vi "Wrapper.vi"(8 "error in (no error)":errorcluster, 10 "Actor in":refnum<class "Actor.lvclass">, 11 "Update gController Data MSG in":refnum<class "Update gController Data MSG.lvclass">) -> (0 "error out":errorcluster, 3 "gController out":refnum<class "gController.lvclass">)   [LabVIEW 2017, in "Controller.lvlib" / "Update gController Data MSG.lvclass"]
uses:
  Update gController Data MSG.lvclass
  C:/Program Files (x86)/National Instruments/LabVIEW 2017/vi.lib/MSR Consulting, LLC/General Reuse/Generic Update Data MSG/Generic Update Data MSG.lvclass
  gController.lvclass
  C:/Program Files (x86)/National Instruments/LabVIEW 2017/vi.lib/MSR Consulting, LLC/General Reuse/SuperActor/SuperActor.lvclass
  <vilib>/ActorFramework/Actor/Actor.lvclass
  gController.lvclass/gController.ctl
  <vilib>/MSR Consulting, LLC/General Reuse/SuperActor/SuperActor.lvclass/SuperActor.ctl
  <vilib>/MSR Consulting, LLC/General Reuse/Generic Update Data MSG/Generic Update Data MSG.lvclass/Generic Update Data MSG.ctl
  <vilib>/MSR Consulting, LLC/General Reuse/Generic Update Data MSG/Read Data.vi
  <vilib>/MSR Consulting, LLC/General Reuse/Generic Update Data MSG/Read ID.vi
  Read DataMap.vi
  <vilib>/MSR Consulting, LLC/General Reuse/SuperActor/Read Log Session.vi
  <vilib>/MSR Consulting, LLC/General Reuse/Data/Data.lvclass
  <vilib>/MSR Consulting, LLC/General Reuse/Session APIs/_Session Fwk/Session - Root.lvclass
  <vilib>/MSR Consulting, LLC/General Reuse/Session APIs/Session Log/System Log.lvclass
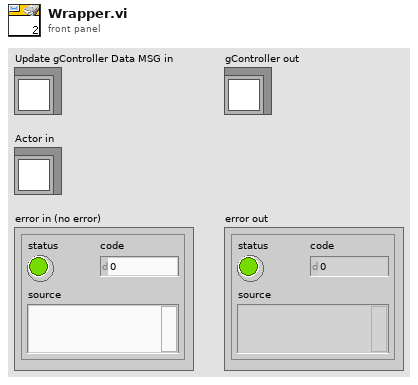
[diagram p1: front panel]
types:
  T1 = typedef "Session - Root.lvclass/Session Handle.ctl" = refnum<data-value>
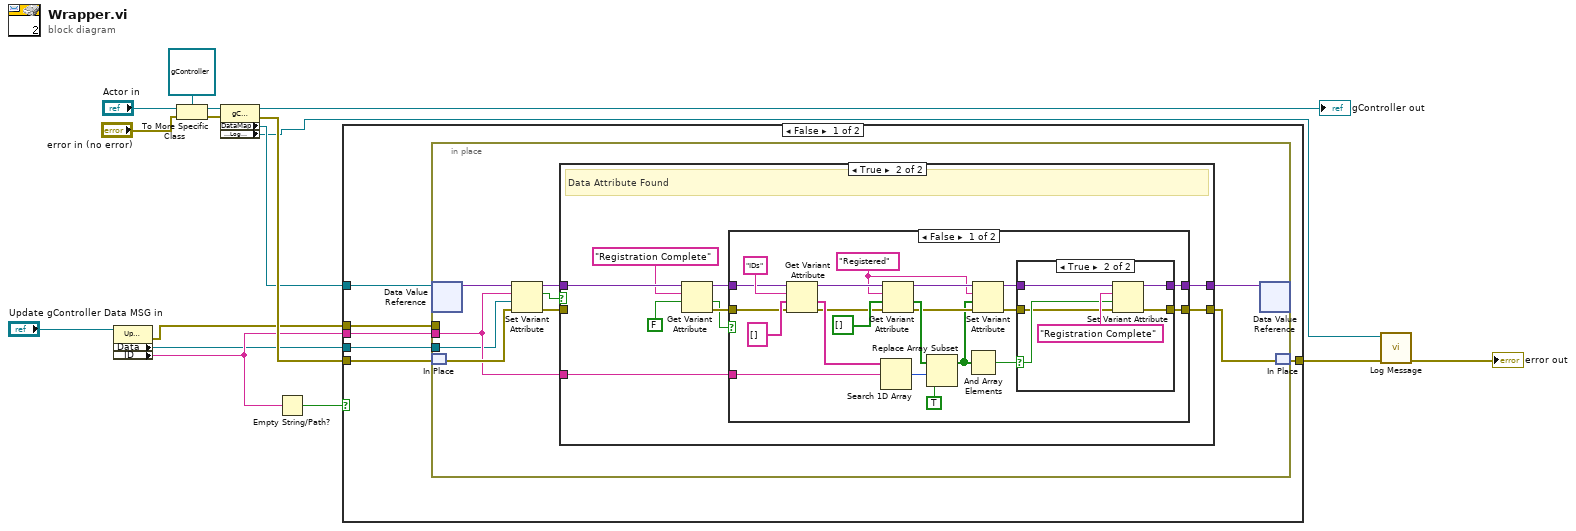
[diagram p0: block diagram]
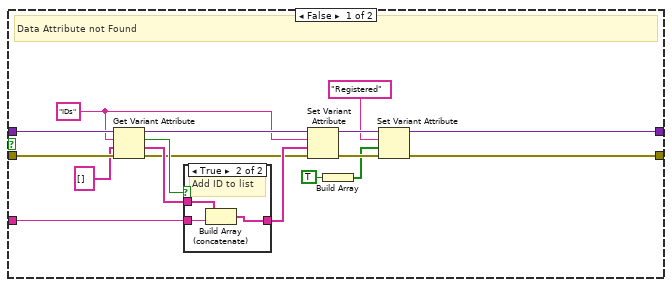
[diagram p2: hidden frame]
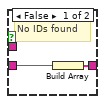
[diagram p3: hidden frame]
diagram:
  n1 = property class="Update gController Data MSG.lvc"(reference="Update gController Data MSG in") -> (error out=w5:errorcluster, "Data"=w4:refnum<class "Data.lvclass">, "ID"=w6:string)  [unwired: 1 in, 1 out]
  n2 = To More Specific Class(target class=refnum<class "gController.lvclass"> refnum ("Controller.lvlib:gController"), reference="Actor in", error in="error in (no error)") -> (specific class reference=w11:refnum<class "gController.lvclass">, error out=w15:errorcluster)
  n3 = property class="gController"(reference=w11, error in=w15) -> (reference out=→"gController out":refnum<class "gController.lvclass">, error out=w16:errorcluster, "DataMap"=w12:refnum<data-value>, "Accessors:Log Session"=w3:T1)
  n4 = Empty String/Path?(string/path=w6) -> (empty?=w8:bool)
  n5 = case shown="False" w8 {
    tunnel: [w22 w94] -> w2
    tunnel: w16 -> [w21 w94]
    tunnel: w6 -> [w20 _]
    tunnel: w5 -> [w19 _]
    tunnel: w12 -> [w18 _]
    tunnel: w4 -> [w17 _]
    frame False {
      n6 = in-place {
        in-place-border: w19 -> [_]
        in-place-border: w20 -> [w26]
        in-place-border: w17 -> [w23]
        n7 = in-place-dvr #1(w18) -> (w29:variant)  [unwired: 1 out]
        n8 = in-place-match #2(w21) -> (w27:errorcluster)
        n9 = Set Variant Attribute(Variant=w29, name=w26, value=w23, error in=w27) -> (Variant out=w31:variant, replaced=w30:bool, error out=w28:errorcluster)
        n10 = case shown="True" w30 {
          tunnel: w31 -> [w48 w60]
          tunnel: w26 -> [w47 w61]
          tunnel: [w45 w62] -> w24
          tunnel: w28 -> [w46 _]
          tunnel: [w44 w55] -> w25
          frame False {
            w41 = "IDs" ("name")
            # "Data Attribute not Found"
            n11 = Get Variant Attribute(Variant=w48, name=w41, default value (empty Variant)=string[] [], error in=w46) -> (duplicate Variant=w42:variant, found=w40:bool, value=w39:string[], error out=w37:errorcluster)
            n12 = case shown="True" w40 {
              tunnel: w39 -> [_ w53]
              tunnel: w47 -> [w50 w52]
              tunnel: [w49 w51] -> w38
              frame False {
                # "No IDs found"
                n13 = Build Array(w50) -> (w49:string[])
              }
              frame True {
                # "Add ID to list"
                n14 = Build Array (concatenate)(w53, w52) -> (w51:string[])
              }
            }
            n15 = Set Variant Attribute(Variant=w42, name=w41, value=w38, error in=w37) -> (Variant out=w36:variant, error out=w35:errorcluster)  [unwired: 1 out]
            n16 = Build Array(TRUE) -> (w32:bool[])
            n17 = Set Variant Attribute(Variant=w36, name="Registered", value=w32, error in=w35) -> (Variant out=w45:variant, error out=w44:errorcluster)  [unwired: 1 out]
          }
          frame True {
            # "Data Attribute Found"
            n18 = Get Variant Attribute(Variant=w60, name="Registration Complete", default value (empty Variant)=FALSE) -> (duplicate Variant=w57:variant, value=w54:bool, error out=w56:errorcluster)  [unwired: 1 in, 1 out]
            n19 = case shown="False" w54 {
              tunnel: [w66 w93] -> w62
              tunnel: w61 -> [w80 _]
              tunnel: w57 -> [w78 w93]
              tunnel: w56 -> [w77 w92]
              tunnel: [w64 w92] -> w55
              frame False {
                w69 = "Registered" ("name")
                n20 = Get Variant Attribute(Variant=w78, name="IDs", default value (empty Variant)=string[] [], error in=w77) -> (duplicate Variant=w79:variant, value=w81:string[], error out=w63:errorcluster)  [unwired: 1 out]
                n21 = Search 1D Array(1D array=w81, element=w80) -> (index of element=w74:i32)  [unwired: 1 in]
                n22 = Get Variant Attribute(Variant=w79, name=w69, default value (empty Variant)=bool[] [], error in=w63) -> (duplicate Variant=w72:variant, value=w75:bool[], error out=w71:errorcluster)  [unwired: 1 out]
                n23 = Replace Array Subset(array=w75, new element=TRUE ("new element/subarray"), index=w74) -> (w70:bool[])
                n24 = And Array Elements(Boolean array=w70) -> (logical AND=w67:bool)
                n25 = Set Variant Attribute(Variant=w72, name=w69, value=w70, error in=w71) -> (Variant out=w68:variant, error out=w65:errorcluster)  [unwired: 1 out]
                n26 = case shown="True" w67 {
                  selector: w67 -> [_ w89]
                  tunnel: w68 -> [w85 w91]
                  tunnel: [w85 w88] -> w66
                  tunnel: w65 -> [w84 w87]
                  tunnel: [w84 w86] -> w64
                  frame False {
                  }
                  frame True {
                    n27 = Set Variant Attribute(Variant=w91, name="Registration Complete", value=w89, error in=w87) -> (Variant out=w88:variant, error out=w86:errorcluster)  [unwired: 1 out]
                  }
                }
              }
              frame True {
              }
            }
          }
        }
        n28 = in-place-dvr #1(w24) -> ()  [unwired: 2 out]
        n29 = in-place-match #2(w25) -> (w22:errorcluster)
      }
    }
    frame True {
    }
  }
  n30 = call <vilib>:"Log Message.vi"("error in"=w2, "session in"=w3) -> ("error out"=→"error out":errorcluster)  [unwired: 8 in, 1 out]
